vi "getLN2Level.vi"(8 "error in (no error)":errorcluster, 11 "Instrument.Oxford1820 in":refnum<class "Instrument.Oxford1820.lvclass">) -> (0 "error out":errorcluster, 2 "LN2 Level (%)":dbl, 3 "Instrument.Oxford1820 out":refnum<class "Instrument.Oxford1820.lvclass">)   [LabVIEW 2019, in "Instrument.Oxford1820.lvclass"]
uses:
  Instrument.Oxford1820.lvclass
  Typedefs/Instrument.Oxford1820.publicCommands-enum.ctl
  Typedefs/getLN2Level--Cluster.ctl
  66ac6e8b-e8b4-4fa9-a84b-b38ed2eef812.vi
  66ac6e8b-e8b4-4fa9-a84b-b38ed2eef812.vi/bc4b1113-a823-458e-8565-88edeb87dfd8.vi
  66ac6e8b-e8b4-4fa9-a84b-b38ed2eef812.vi/18188d71-6a79-4892-b802-91496138f2a2.vi
  <vilib>/Utility/Data Type/Get Type Information.vi
  <vilib>/JDP Science/JSONtext/JSON text to Variant.vi
  <vilib>/JDP Science/JSONtext/LVClass Serializer/JSONtext LVClass Serializer.lvclass
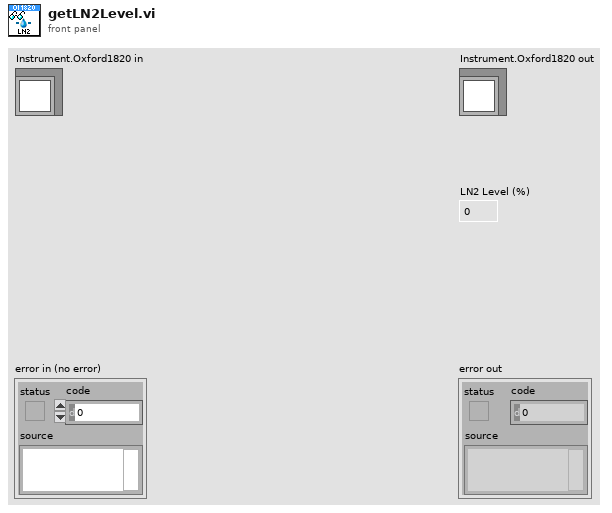
[diagram p1: front panel]
types:
  T1 = typedef "Instrument.Oxford1820.lvclass/getLN2Level--Cluster.ctl" = cluster{"LN2Level":dbl}
  T2 = typedef "Instrument.Oxford1820.lvclass/Instrument.Oxford1820.publicCommands-enum.ctl" = enum16{"setMagnet", "getMagnet", "getMagnetTarget", "getLHeLevel", "getLN2level"}
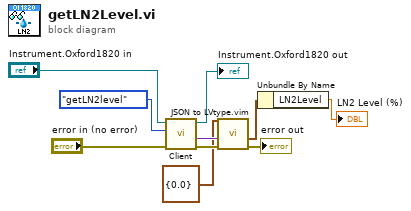
[diagram p0: block diagram]
diagram:
  n1 = call-dynamic "Client.vi"("error in (no error)"="error in (no error)", "Command in"=Instrument.Oxford1820.publicCommands-enum."getLN2level" ("publicCommands"), "Instrument in"="Instrument.Oxford1820 in") -> ("error out"=w6:errorcluster, "Data out"=w5:variant, "Instrument out"=→"Instrument.Oxford1820 out":refnum<class "Instrument.Oxford1820.lvclass">)  [unwired: 5 in, 1 out]
  n2 = call "JSON to LVtype.vim"("type"=T1 {"LN2Level"=0.0} ("getN2Level"), "error in (no error)"=w6, "JSON Data in"=w5) -> ("error out"=→"error out":errorcluster, "Data out"=w2:T1)  [unwired: 7 in]
  n3 = Unbundle By Name(w2) -> ("LN2Level"=→"LN2 Level (%)":dbl)
